vi "GetPackages.vi"(11 "IcmMessageService in":refnum<class "IcmMessageService.lvclass">) -> (0 "IcmMessageService in 2":refnum<class "IcmMessageService.lvclass">, 1 "string":string)   [LabVIEW 2016]
uses:
  <vilib>/addons/InsightCM/MessageBus/MessageService/IcmMessageService.lvclass
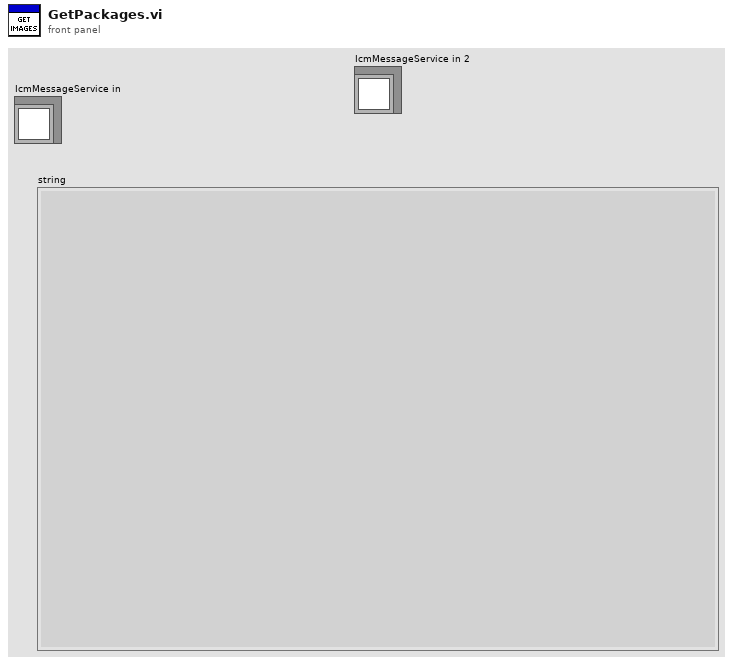
[diagram p1: front panel]
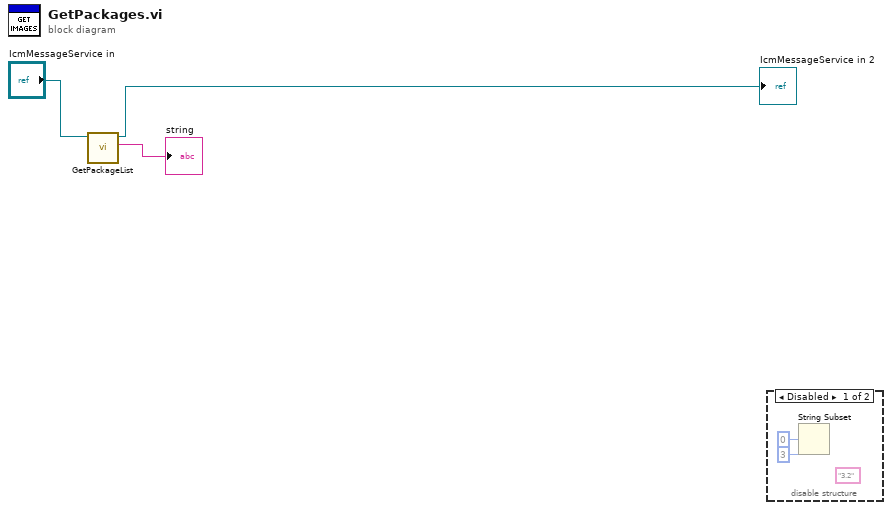
[diagram p0: block diagram]
diagram:
  n1 = call "GetPackageList.vi"("service"="IcmMessageService in") -> ("string"=→"string":string, "service out"=→"IcmMessageService in 2":refnum<class "IcmMessageService.lvclass">)  [unwired: 8 in, 1 out]
  n2 = disable-structure shown="Disabled" {
    frame Disabled {
      (unwired) "3.2" ("y")
      n3 = String Subset(offset (0)=0, length (rest)=3 ("length (rest)")) -> (substring=w6:string)  [unwired: 1 in]
    }
    frame Enabled {
    }
  }
